vi "MAIN_VI.vi"() -> ()   [LabVIEW 2017]
doc: "This Vi is used for Testing CAN TX RX for Any Project its General VI for CAN TESTING"
uses:
  Control 1.ctl
  CAN TESTING CLUSTER.ctl
  CAN_OPERATION _TYPEDEF.ctl
panel:
  in  "Default ID 3":u32=769 format="%.0x"
  in  "Write/Read 2":bool
  in  "Default ID 2":u32=721 format="%.0x"
  in  "Default ID 1":u32=1111 format="%.0x"
  in  "EXIT":bool
  out "Rx ID":u32 format="%.0x"
  out "Rx Data":u8[](array[numeric]) format="%.0x"
  out "can read array":u32[][](array[numeric])
  in  "DataLength":u32=1
  in  "Write/Read":bool
  out "User_Ack":string
  out "CAN Table":string[][](table)
  in  "Command Name":string(combo)
  in  "CAN Write":bool
  in  "Tx_Message":u8[](array[numeric])=[89, 42, 118, 0, 0, 0, 0, 0] format="%.0x"
  in  "Tx ID":u32=769 format="%.0x"
  in  "Interface":string(combo)="CAN0"
  in  "Baudrate":u32=500000
  out "Error out 2":errorcluster
  in  "Error in 2":errorcluster {"code" format="%.0x"}
  # "CAN TESTING SOFTWARE"
  # "4F9"
  # "ver 1.1.1"
  # "CAN MONITOR"
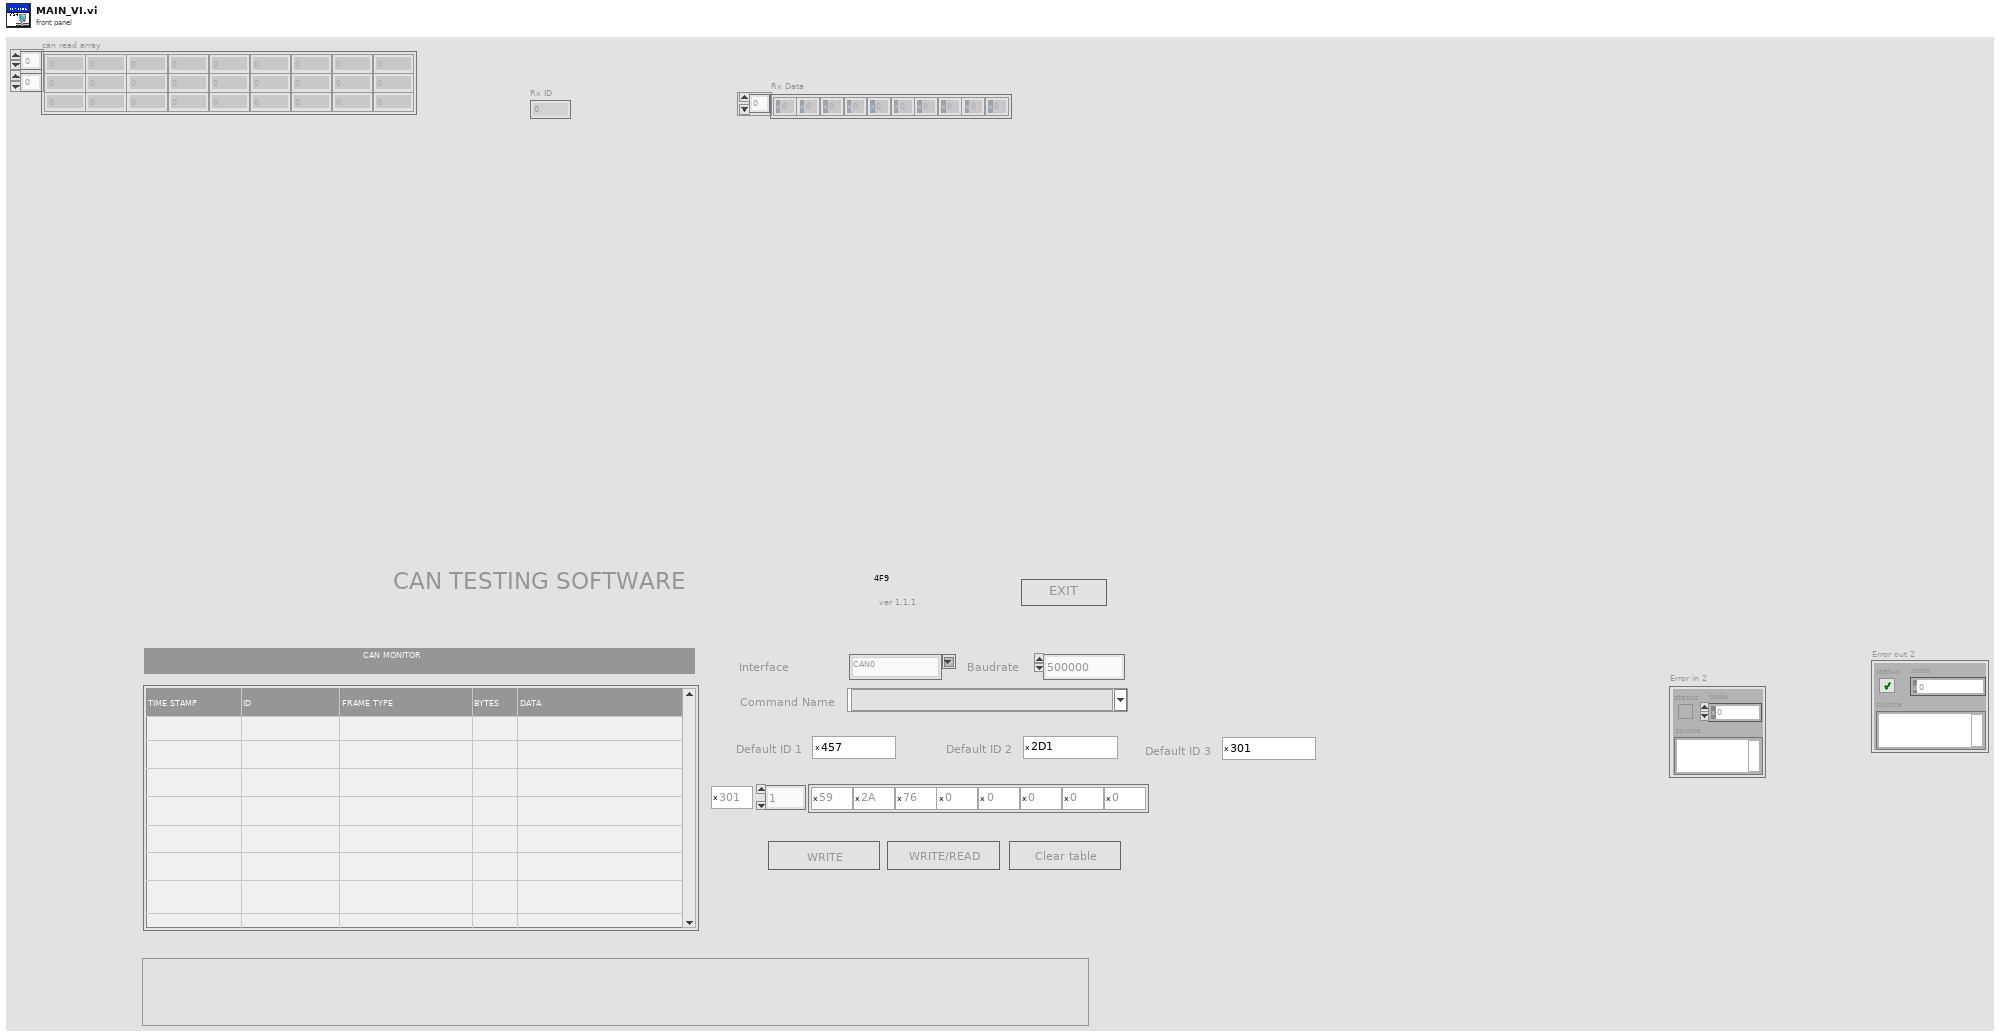
[diagram p1: front panel]
types:
  T1 = typedef "CAN TESTING CLUSTER.ctl" = cluster{"User_Ack":string, "Command Name":string, "Tx_Message":u32[], "Tx_ID":u8, "CAN Table":string[][]}
  T2 = typedef "Control 1.ctl" = enum16{"INITIALIZE", "WRITE", "READ", "WRITE/READ", "RESET", "POLL", "CLOSE"}
  T3 = typedef "CAN_OPERATION _TYPEDEF.ctl" = string
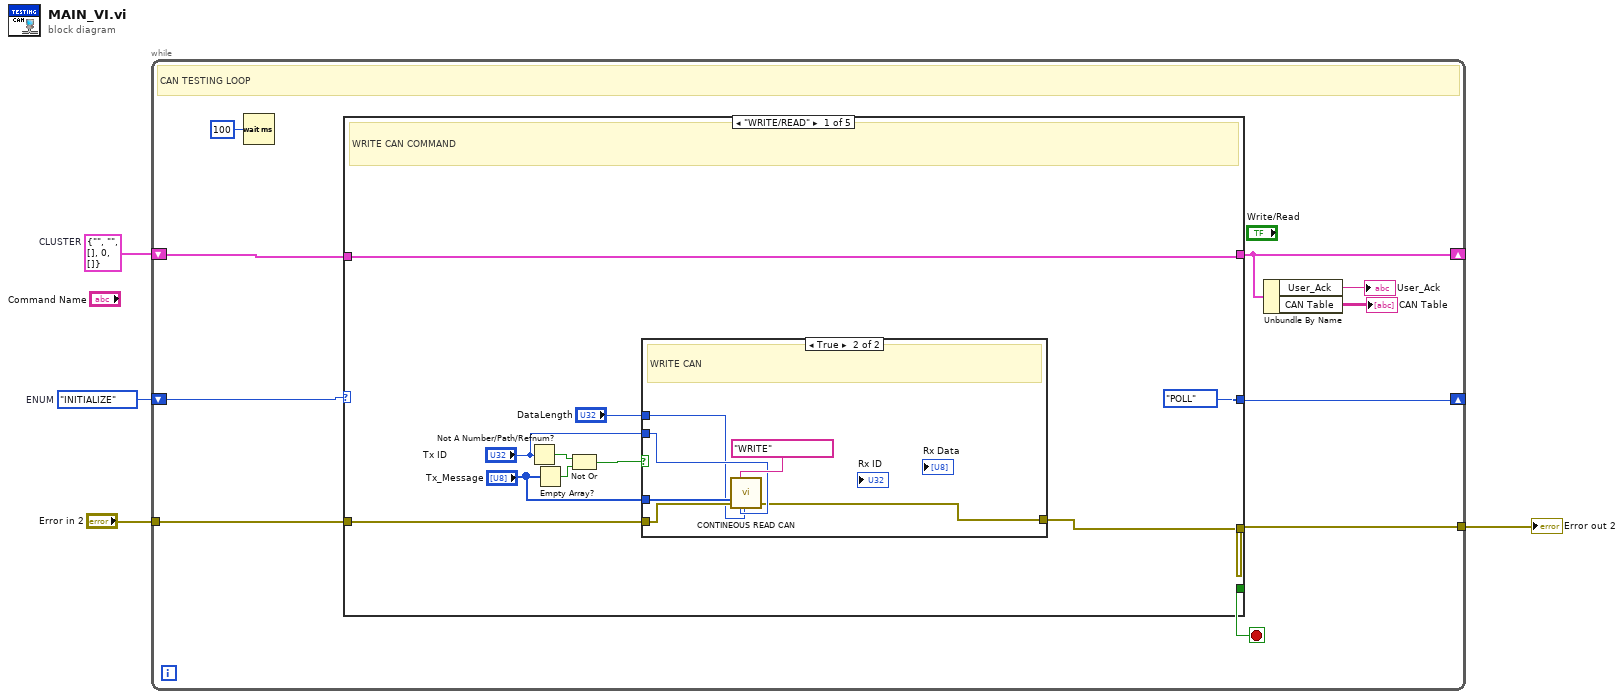
[diagram p0: block diagram]
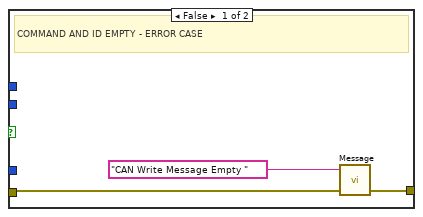
[diagram p2: hidden frame]
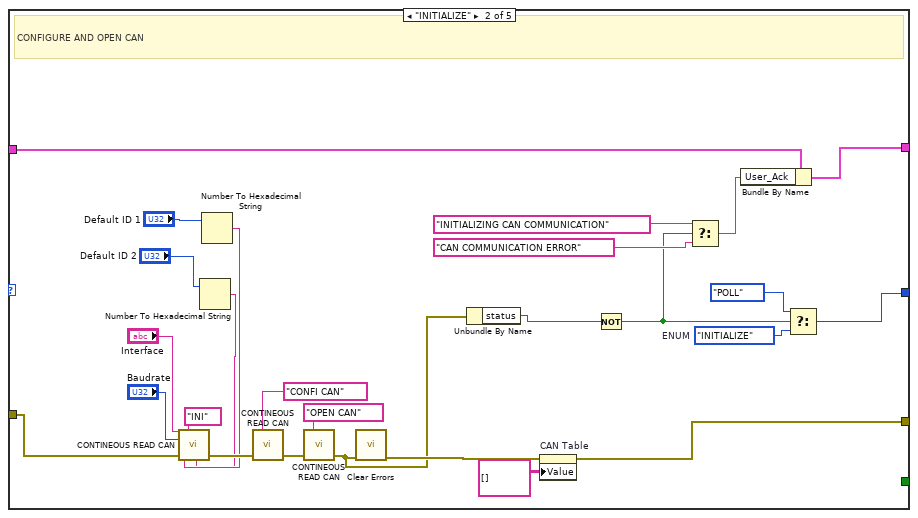
[diagram p3: hidden frame]
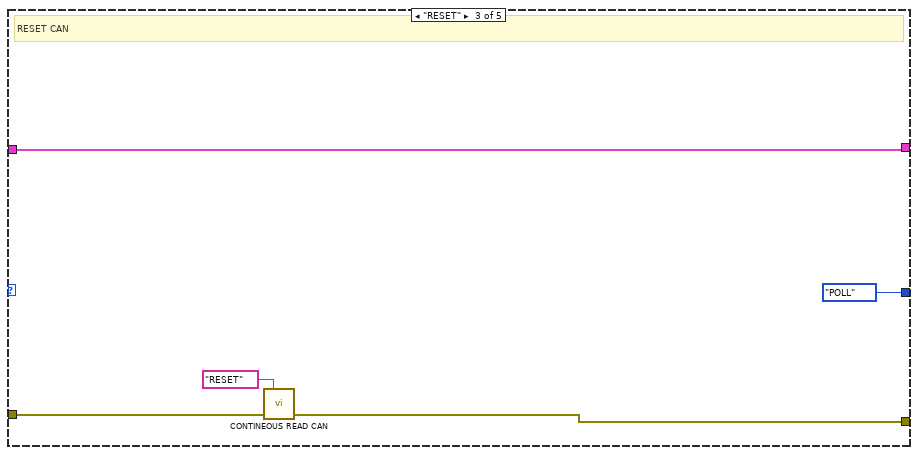
[diagram p4: hidden frame]
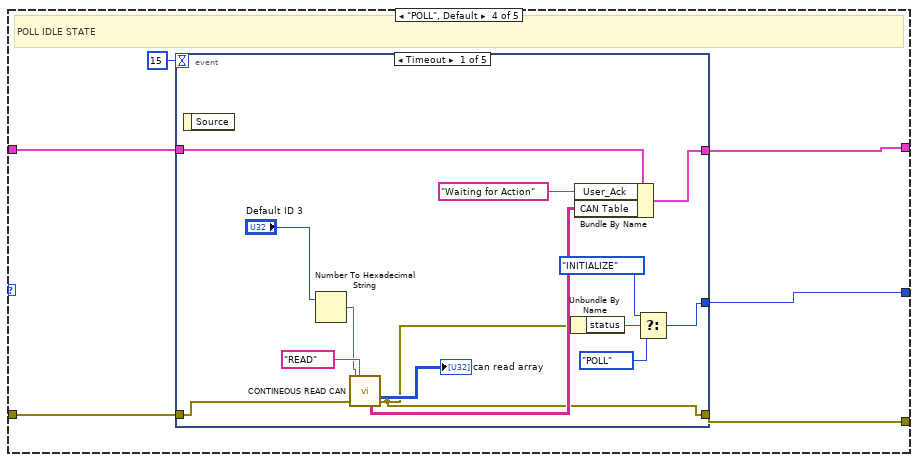
[diagram p5: hidden frame]
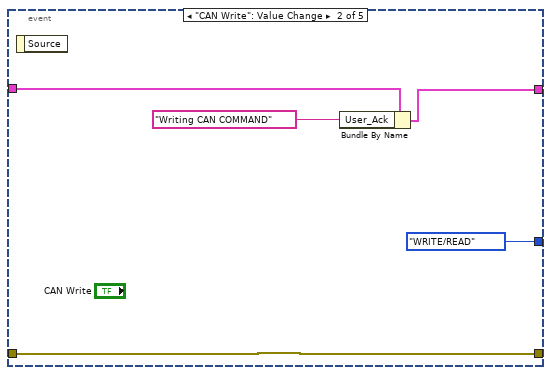
[diagram p6: hidden frame]
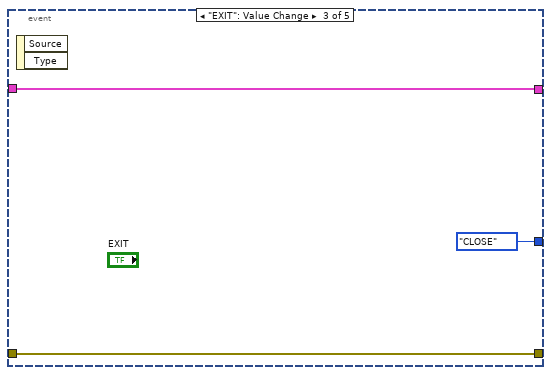
[diagram p7: hidden frame]
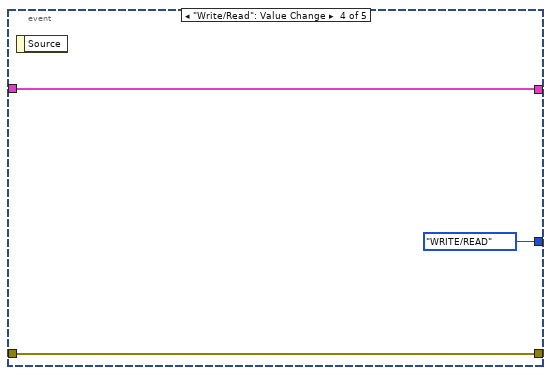
[diagram p8: hidden frame]
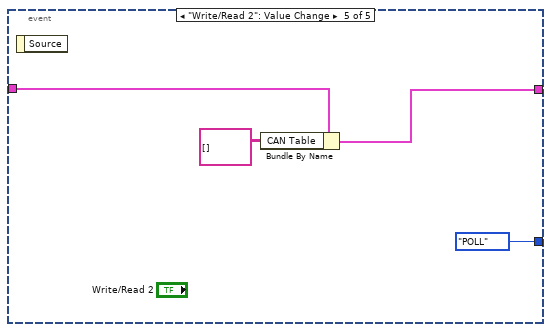
[diagram p9: hidden frame]
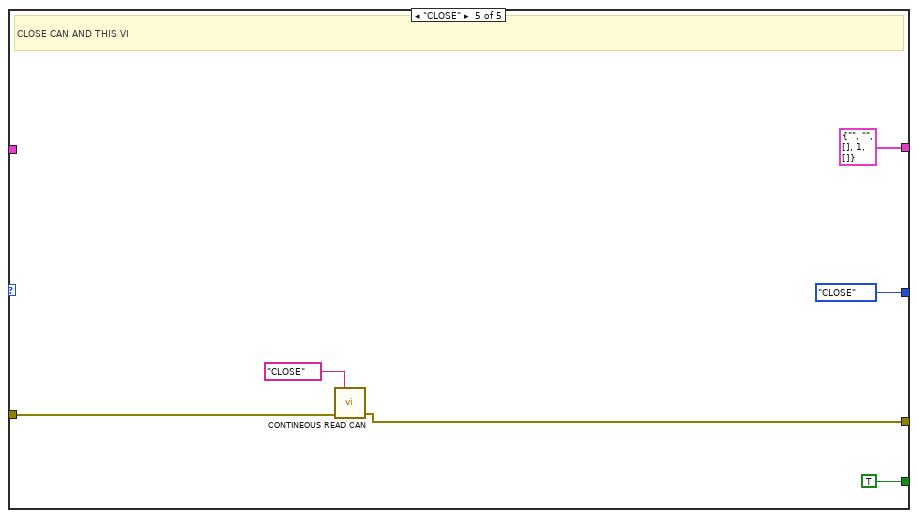
[diagram p10: hidden frame]
diagram:
  w1 = T1 {"User_Ack"="", "Command Name"="", "Tx_Message"=[], "Tx_ID"=0, "CAN Table"=[]}  # CLUSTER
  w3 = Control_1."INITIALIZE"  # ENUM
  n1 = while {
    tunnel: [w14] -> w2
    shift-right: [w9] -> _
    shift-left: w3 -> [w11]
    tunnel: "Error in 2" -> [w10]
    shift-right: [w7] -> _
    shift-left: w1 -> [w8]
    stop <- w13 stop-if-true
    # "CAN TESTING LOOP"
    n2 = Wait (ms)(milliseconds to wait=u32 100) -> ()  [unwired: 1 out]
    n3 = case shown="\"WRITE/READ\"" w11 {
      tunnel: [w24 w53 w63 w65 w103] -> w14
      tunnel: [_ _ _ _ TRUE] -> w13
      tunnel: w10 -> [w20 w41 w62 w66 w104]
      tunnel: [Control_1."POLL" w51 Control_1."POLL" w69 Control_1."CLOSE"] -> w9
      tunnel: [w15 w56 w60 w67 T1 {"User_Ack"="", "Command Name"="", "Tx_Message"=[], "Tx_ID"=1, "CAN Table"=[]}] -> w7
      tunnel: w8 -> [w15 w55 w60 w68 _]
      frame "WRITE/READ" {
        # "WRITE CAN COMMAND"
        n4 = Not A Number/Path/Refnum?(number/path/refnum="Tx ID") -> (NaN/Path/Refnum?=w23:bool)
        n5 = Empty Array?(array="Tx_Message") -> (empty?=w22:bool)
        n6 = Not Or(1:w22, 2:w23) -> (0:w21:bool)
        n7 = case shown="True" w21 {
          tunnel: [w27 w29] -> w24
          tunnel: w20 -> [w25 w30]
          tunnel: "Tx ID" -> [_ w32]
          tunnel: "Tx_Message" -> [_ w31]
          tunnel: "DataLength" -> [_ w28]
          frame False {
            # "COMMAND AND ID EMPTY - ERROR CASE"
            n8 = call "Message.vi"("error in (no error)"=w25, "Message"="CAN Write Message Empty ") -> ("error out"=w27:errorcluster)  [unwired: 3 in]
          }
          frame True {
            # "WRITE CAN"
            n9 = call "CONTINEOUS READ CAN.vi"("WRITE CMD"=w31, "Error in 2"=w30, "CAN OPERATION"="WRITE", "WRITE AR ID"=w32, "DataLength"=w28) -> ("Error out 2"=w29:errorcluster)  [unwired: 16 in, 6 out]
          }
        }
      }
      frame "INITIALIZE" {
        w50 = Control_1."INITIALIZE"  # ENUM
        # "CONFIGURE AND OPEN CAN"
        n10 = Number To Hexadecimal String(2:"Default ID 2") -> (0:w34:string)  [unwired: 1 in]
        n11 = Number To Hexadecimal String(2:"Default ID 1") -> (0:w35:string)  [unwired: 1 in]
        n12 = call "CONTINEOUS READ CAN.vi"("interface"="Interface", "Baudrate"="Baudrate", "Error in 2"=w41, "Default ID 1"=w35, "CAN OPERATION"=T3 "INI", "Default ID 2"=w34) -> ("Error out 2"=w42:errorcluster)  [unwired: 15 in, 6 out]
        n13 = call "CONTINEOUS READ CAN.vi"("Error in 2"=w42, "CAN OPERATION"="CONFI CAN") -> ("Error out 2"=w57:errorcluster)  [unwired: 19 in, 6 out]
        n14 = call "CONTINEOUS READ CAN.vi"("Error in 2"=w57, "CAN OPERATION"="OPEN CAN") -> ("Error out 2"=w49:errorcluster)  [unwired: 19 in, 6 out]
        n15 = call <vilib>:"Clear Errors.vi"("error in (no error)"=w49) -> ("error out"=w54:errorcluster)  [unwired: 5 in, 1 out]
        n16 = Unbundle By Name(w49) -> ("status"=w43:bool)
        n17 = property on="CAN Table" class="Tbl (strict)"(error in=w54, "Value"=string[][] [] ("CAN Table")) -> (error out=w53:errorcluster)  [unwired: 1 in, 1 out]
        n18 = Not(x=w43) -> (.not. x?=w46:bool)
        n19 = Select(t="INITIALIZING CAN COMMUNICATION" ("User_Ack"), s=w46, f="CAN COMMUNICATION ERROR" ("User_Ack")) -> (s? t:f=w45:string)
        n20 = Bundle By Name(cluster=w55, "User_Ack"=w45) -> (w56:T1)
        n21 = Select(t=Control_1."POLL", s=w46, f=w50) -> (s? t:f=w51:T2)
      }
      frame "RESET" {
        # "RESET CAN"
        n22 = call "CONTINEOUS READ CAN.vi"("Error in 2"=w62, "CAN OPERATION"=T3 "RESET") -> ("Error out 2"=w63:errorcluster)  [unwired: 19 in, 6 out]
      }
      frame "POLL", Default {
        # "POLL IDLE STATE"
        n23 = event shown="[0] Timeout" {
          selector: _ -> [_ _ _ _ _]
          dyn-events: _ -> [_ _ _ _ _]
          timeout: 15 -> [_ _ _ _ _]
          tunnel: [w74 Control_1."WRITE/READ" Control_1."CLOSE" Control_1."WRITE/READ" Control_1."POLL"] -> w69
          tunnel: w68 -> [w84 w88 w90 w94 w98]
          tunnel: [w83 w87 w90 w94 w97] -> w67
          tunnel: w66 -> [w79 w85 w91 w93 _]
          tunnel: [w77 w85 w91 w93 _] -> w65
          event Timeout {
            n24 = event-data() -> ()  [unwired: 1 in, 1 out]
            n25 = Number To Hexadecimal String(2:"Default ID 3") -> (0:w71:string)  [unwired: 1 in]
            n26 = call "CONTINEOUS READ CAN.vi"("Error in 2"=w79, "Default 3"=w71, "CAN OPERATION"="READ") -> ("Actual CAN Array"=w80:string[][], "can read array"=→"can read array":u32[][], "Error out 2"=w77:errorcluster)  [unwired: 18 in, 4 out]
            n27 = Unbundle By Name(w77) -> ("status"=w76:bool)
            n28 = Bundle By Name(cluster=w84, "User_Ack"="Waiting for Action", "CAN Table"=w80) -> (w83:T1)
            n29 = Select(t=Control_1."INITIALIZE", s=w76, f=Control_1."POLL") -> (s? t:f=w74:T2)
          }
          event "CAN Write": Value Change {
            n30 = event-data() -> ()  [unwired: 1 in, 1 out]
            n31 = Bundle By Name(cluster=w88, "User_Ack"="Writing CAN COMMAND") -> (w87:T1)
          }
          event "EXIT": Value Change {
            n32 = event-data() -> ()  [unwired: 1 in, 2 out]
          }
          event "Write/Read": Value Change {
            n33 = event-data() -> ()  [unwired: 1 in, 1 out]
          }
          event "Write/Read 2": Value Change {
            n34 = event-data() -> ()  [unwired: 1 in, 1 out]
            n35 = Bundle By Name(cluster=w98, "CAN Table"=string[][] []) -> (w97:T1)
          }
        }
      }
      frame "CLOSE" {
        # "CLOSE CAN AND THIS VI"
        n36 = call "CONTINEOUS READ CAN.vi"("Error in 2"=w104, "CAN OPERATION"="CLOSE") -> ("Error out 2"=w103:errorcluster)  [unwired: 19 in, 6 out]
      }
    }
    n37 = Unbundle By Name(w7) -> ("User_Ack"=→"User_Ack":string, "CAN Table"=→"CAN Table":string[][])
  }
  "Error out 2" <- w2
